vi "trial 1.vi"() -> ()   [LabVIEW 2013]
panel:
  out "number":i32[](array[numeric])
  out "Array 3":i32[][](array[numeric])
  in  "index":i32
  out "Array 2":i32[][](array[numeric])
  in  "Full transition sequence from service to end":string[](array[string])=["-2 0 3 0 -3 0 4 -4 0\r\n", "0 3\r\n", "0 4 -3 0 -4 1 0 4 -3 0\r\n", "0\r\n", "-2 0 3 -3 0 -4 1 -4 0 3 -3 4 -3 0 2 0 3\r\n", "0 3 0 1\r\n", "0 1 0 3\r\n", "0 3 -2 0 4\r\n", "0\r\n", "0 -3 4 0 2 -2 0 -3 0 3 -2 3 -3 4\r\n", "0 -3 4 -3 0\r\n", "-2 0 -2 2 0\r\n", "0 3 -2\r\n", "0 4 -3 0 3 -2 0 -3 4 -3 0 3 -2 2 -2 0 4 0\r\n", "2 0 1 -4 0 3 0 -4 4 0 -4 4 0 2 0 4 0 -3 4 -3 0 -4 0 4\r\n", "0 4\r\n", "-2 0 -2 0 3 0\r\n", "0 3 0 -2 3\r\n", "0 4 0 4 -4 0 2 0 -4 4 -3 0 -2 2 -2 0 4 -3 0 2 0 3 0\r\n", "0 4 -3 0 1 -1 0 3 0 -2 2 -2 0 -3 4 -3 0 4 -4 1 0\r\n", "", "0 -3\r\n", "2 0 3 0 1 0 -2 3\r\n", "0\r\n", "1 -1 0\r\n", "0 -2 3 0\r\n", "0 1 0 4 0 4 -4 4\r\n", "0 1 -1 0 3\r\n", "0 2 -2 3 -3 4\r\n", "-2 2 0 -2 3\r\n", "0 -1\r\n", "0 4 -4 4 0 3 0 -2 0 -4 0 1 -4\r\n", "-2 0 4 0 -3 3 0 -2 2 -2 0 -4 0 4 0\r\n", "0 -1 0 -4 4 -4 1 -4 0\r\n", "1 -4 1 0 2 0 -3 0 2 0 -2 0 1 0 1 -4 4 -4 1 0 3 -2 0 -4 4 -4\r\n", "0 1 -4 4 -4 1\r\n", "0 3 0 -3 3 0 1 0 1 -4 4\r\n", "0 1 -4 0 1 -4\r\n", "0 3 -2 0 1 -4 1 0 2 0 4 0 4 0 -1 2 -1 0\r\n", "1 0 -1 0 2 0 4 -4\r\n", "-4\r\n", "-1 0 4\r\n", "0 1 -1 0 1 -4 0\r\n", "-1 0 1 -4 0 3 0 2 0 4 0 -4 4 -4 0 -1 0 -4 0 -2 0 4\r\n", "0 4 0\r\n", "0 4 -4 0 2 -1 0 2 0 4 -4 1 -4 4 0 3\r\n", "0 4 0 2 0\r\n", "1 0 -1 1 0 -4 1 -4 1 0 -4\r\n", "0 3 -2 0 -4\r\n", "2 -1 0 -4 4 -4 0 2 0 4\r\n", "1 0\r\n", "-1 0 -1 1 0 -4\r\n", "0 3 0\r\n", "0 -4 4 -4 0 -4 0 4 0 2 0 1 -4 4\r\n", "-1 0 1 -4\r\n", "-1 0 2 -1 0 2\r\n", "1 -1 0 4 -4 1\r\n", "-1 0 1 -4 4 -4 0 -4 4\r\n", "0 3 0 3 0 1 -1 0 1\r\n", "-1 0 4 0 4 -4 1 0 -4 0\r\n", "1 0 4\r\n", "0 -1 0 2 -1 0 -2 3 -2 0 -4 4 -4\r\n", "0 3 0\r\n", "2 -1 0 1 -4 4 -4 0 2 0\r\n", "0 4 -4 1 0 1 0 1 -4 0 2 0 4 0 4 -4 1\r\n", "1 -1 0 3 0 3 0 1 0 4\r\n", "0 -4 0 -2 0 -4\r\n", "0 -4 4 -4 0 -2 0 2 0\r\n", "-1 0 4 -4 0\r\n", "1 0 -1 2 0 4\r\n", "0 2 0 -2 0\r\n", "0 1 -4 0 -4 0 3 -2 0 -4 0 -4 4 -4 1\r\n", "0 4 0 4 0 4 0 4 0 -2 3 0 3 0 4 0\r\n", "-4 -1\r\n", "-2 0 1 0 -4 4\r\n", "0 4\r\n", "-2 2 0 -1 -4 1 0 3 0\r\n", "-1 0 -1 2\r\n", "0 -1 1 0 4 0 3 -2 0 -2 3 -2 0 4 0 -2 2\r\n", "2 -1 0 4\r\n", "0 4 0 2 0 -2 0\r\n", "1 -1 0 3 0 -4 4 -4 0\r\n", "2 -1 0 3 -2 0 -3 0 3 0 -3 0\r\n", "0 4 0 4 -4 1 -1 0 -3 0 1 -4 1 0 4 0 -4 0 -4 4 -4 1\r\n", "0 -4 1 0 -4 4\r\n", "0 4 0 -2 2 -2 2 -2 2\r\n", "-2 2 -1 0 4 0 2 0 4 0 2 -2 0 4\r\n", "1 0 -1 0 -1 0 1 -1\r\n", "-2 2 -2 3\r\n", "1 0 -1 0 -1 2 0 2 -2 0 -4 0\r\n", "-2 2 0 3 -2 2\r\n", "0\r\n", "1 -1 0 3\r\n", "0 4 0\r\n", "-2 0 1 -4 0 -3 0\r\n", "1 0 -1 2 -1 1 -4\r\n", "0 4\r\n", "-2 0 -1 1\r\n", "0 3 0 3 0 3 -2\r\n", "-4 0 -4 4\r\n", "0 4 0 -4 0 -4\r\n", "-2 2 0 4 -4 0 2 -2\r\n", "-2 2 -2 0 -1\r\n", "0 4 -3 0\r\n", "0 1 0 -1 1\r\n", "-4 0\r\n", "-2 0 3 0 1 0 3 -2 0 -1 0 4 0 3 0 -3 3 -3\r\n", "0 4 0 -2 0 1 0 -4 4 -3 0 1 0 4 0 -4 1 0 3 -3 0\r\n", "0 -1 2\r\n", "2 0 -3 4 0\r\n", "-4 0 -3 3 -3 0 -3 3 0 -2 3 0\r\n", "0 -1 1 -4 4 -3 0 3 0\r\n", "0 -1 2 0 3 0 1 -4 4 0 2 0\r\n", "2 -2 0 -4 0 -4 4 0 -4\r\n", "1 -1 2 -1\r\n", "2 0 -2 0 4 0 2 0 3 0 -2 0 -4\r\n", "1 -1 0 -1\r\n", "0 1 -4 1\r\n", "0 4 0 -1 1 -1 0\r\n", "0 3\r\n", "-2 0\r\n", "1 -4 0 -2 0 4 0 -4 0 4 -3 0 1 -4 0 1\r\n", "0 -3 3 -2 0 3 0 -2 2\r\n", "1 0\r\n", "2\r\n", "0 -4\r\n", "0 4 0 -4 0 -3 3 -3 0 -2 0 -2 0 4 0 -1 1 0 3 0 -4 1 -4 0 4\r\n", "2 0 -1 1\r\n", "0 2 0 4 0 4 -4 0 -1 2\r\n", "0 3 -2 0 3 -2\r\n", "1 0 -3 3 0 -4\r\n", "0 -3 3 0 -1 0\r\n", "2 -2 0 1\r\n", "-4 1 -4 1 -4 0\r\n", "0 4 0 2 0 -4 1 2 -1 0 4 0 1 0 4 -4 4 0 -4 4 0\r\n", "-2 0 3 0 -2 0\r\n"]
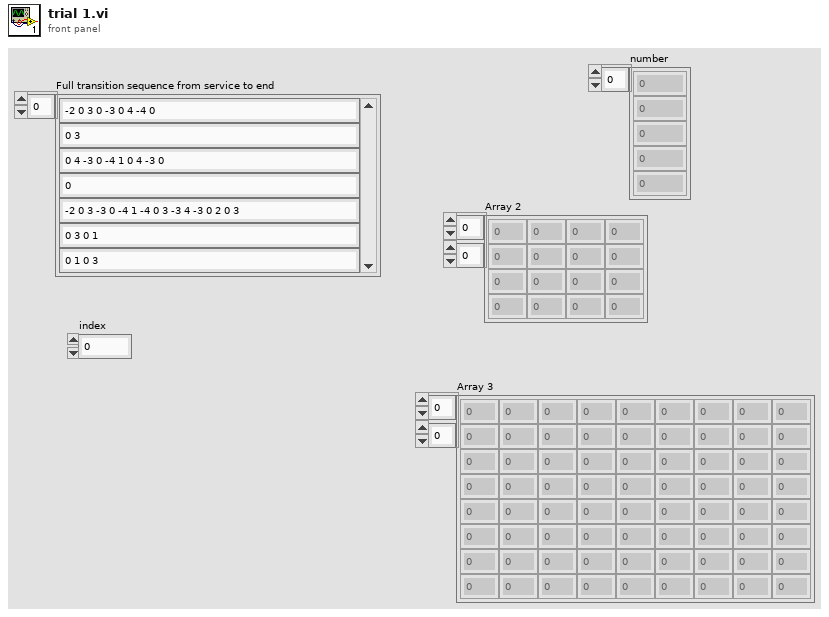
[diagram p1: front panel]
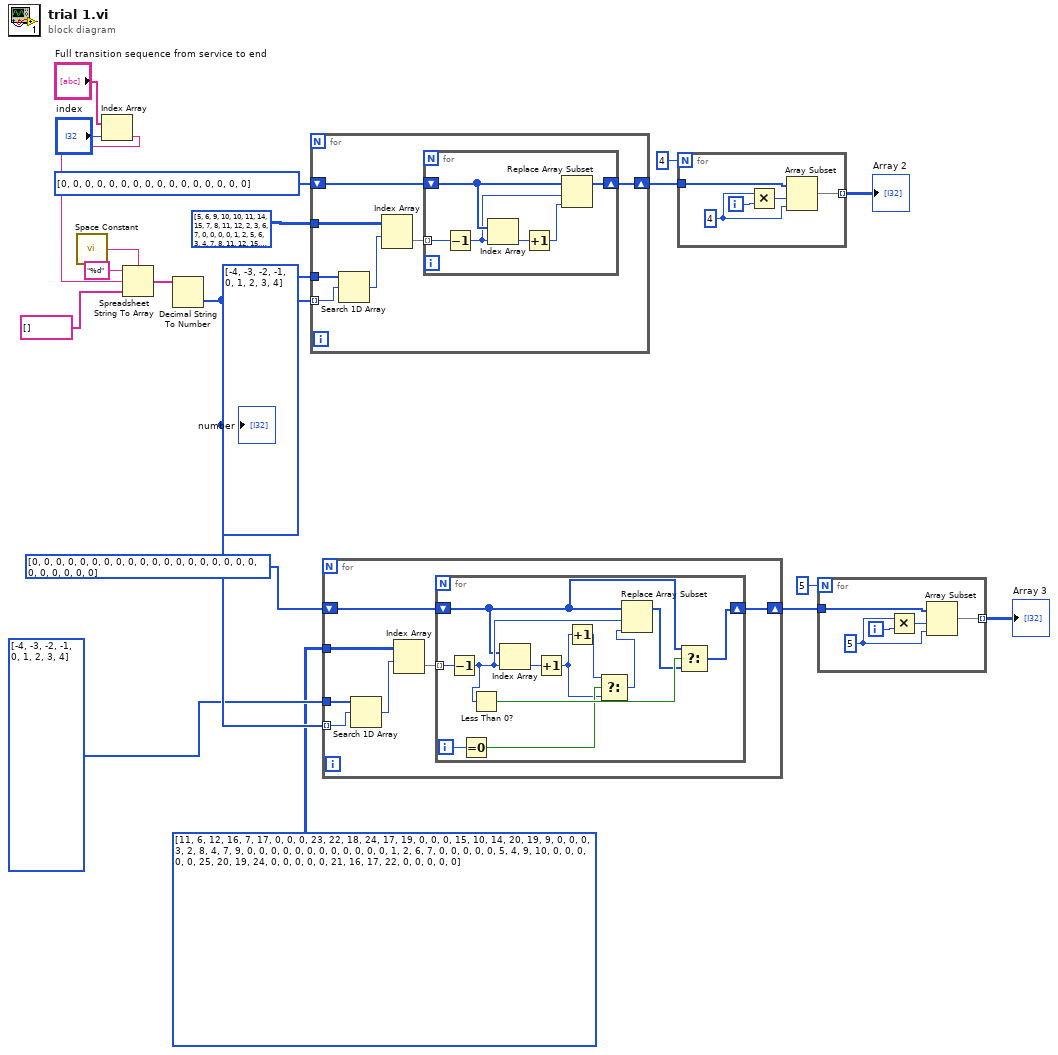
[diagram p0: block diagram]
diagram:
  n1 = call <vilib>:"Space Constant.vi"() -> ("String"=w20:string)
  n2 = Index Array(array="Full transition sequence from service to end", index="index") -> (element=w9:string)
  n3 = Spreadsheet String To Array(delimiter (Tab)=w20, format string="%d", spreadsheet string=w9, array type (2D Dbl)=string[] []) -> (array=w17:string[])
  n4 = Decimal String To Number(string=w17) -> (number=w4:i32[])  [unwired: 2 in, 1 out]
  "number" <- w4
  n5 = for {
    tunnel: w4 -> [w26] mode=indexing
    tunnel: i32[] [-4, -3, -2, -1, 0, 1, 2, 3, 4] ("deleted portion") -> [w27]
    tunnel: i32[][] [[5, 6, 9, 10], [10, 11, 14, 15], [7, 8, 11, 12], [2, 3, 6, 7], [0, 0, 0, 0], [1, 2, 5, 6], [3, 4, 7, 8], [11, 12, 15, 16], [9, 10, 13, 14]] ("array w/ subset deleted") -> [w25]
    shift-right: [w21] -> w13
    shift-left: i32[] [0, 0, 0, 0, 0, 0, 0, 0, 0, 0, 0, 0, 0, 0, 0, 0] -> [w22]
    n6 = Search 1D Array(1D array=w27, element=w26) -> (index of element=w24:i32)  [unwired: 1 in]
    n7 = Index Array(array=w25, index (row)=w24) -> (element=w23:i32[])  [unwired: 1 in]
    n8 = for {
      tunnel: w23 -> [w29] mode=indexing
      shift-right: [w30] -> w21
      shift-left: w22 -> [w32]
      n9 = Decrement(x=w29) -> (x-1=w28:i32)
      n10 = Index Array(array=w32, index=w28) -> (element=w33:i32)
      n11 = Increment(x=w33) -> (x+1=w31:i32)
      n12 = Replace Array Subset(array=w32, new element=w31, index=w28) -> (w30:i32[])
    }
  }
  n13 = for {
    tunnel: w4 -> [w39] mode=indexing
    tunnel: i32[] [-4, -3, -2, -1, 0, 1, 2, 3, 4] ("deleted portion") -> [w40]
    tunnel: i32[][] [[11, 6, 12, 16, 7, 17, 0, 0, 0], [23, 22, 18, 24, 17, 19, 0, 0, 0], [15, 10, 14, 20, 19, 9, 0, 0, 0], [3, 2, 8, 4, 7, 9, 0, 0, 0], [0, 0, 0, 0, 0, 0, 0, 0, 0], [1, 2, 6, 7, 0, 0, 0, 0, 0], [5, 4, 9, 10, 0, 0, 0, 0, 0], [25, 20, 19, 24, 0, 0, 0, 0, 0], [21, 16, 17, 22, 0, 0, 0, 0, 0]] ("array w/ subset deleted") -> [w38]
    shift-right: [w34] -> w5
    shift-left: i32[] [0, 0, 0, 0, 0, 0, 0, 0, 0, 0, 0, 0, 0, 0, 0, 0, 0, 0, 0, 0, 0, 0, 0, 0, 0] -> [w35]
    n14 = Search 1D Array(1D array=w40, element=w39) -> (index of element=w37:i32)  [unwired: 1 in]
    n15 = Index Array(array=w38, index (row)=w37) -> (element=w36:i32[])  [unwired: 1 in]
    n16 = for {
      tunnel: w36 -> [w51] mode=indexing
      shift-right: [w45] -> w34
      shift-left: w35 -> [w47]
      i -> [w50]
      n17 = Decrement(x=w51) -> (x-1=w49:i32)
      n18 = Equal To 0?(x=w50) -> (x = 0?=w44:bool)
      n19 = Less Than 0?(x=w49) -> (x < 0?=w48:bool)
      n20 = Index Array(array=w47, index=w49) -> (element=w52:i32)
      n21 = Increment(x=w52) -> (x+1=w42:i32)
      n22 = Increment(x=w42) -> (x+1=w41:i32)
      n23 = Select(t=w41, s=w44, f=w42) -> (s? t:f=w43:i32)
      n24 = Replace Array Subset(array=w47, new element=w43, index=w49) -> (w46:i32[])
      n25 = Select(t=w47, s=w48, f=w46) -> (s? t:f=w45:i32[])
    }
  }
  n26 = for {
    N: 4 -> [_]
    tunnel: w13 -> [w57]
    tunnel: [w53] -> w11 mode=indexing
    i -> [w56]
    w55 = 4 ("length")
    n27 = Multiply(x=w55, y=w56) -> (x*y=w54:i32)
    n28 = Array Subset(array=w57, index=w54, length=w55) -> (w53:i32[])
  }
  "Array 2" <- w11
  n29 = for {
    N: 5 -> [_]
    tunnel: w5 -> [w62]
    tunnel: [w58] -> w7 mode=indexing
    i -> [w61]
    w60 = 5 ("length")
    n30 = Multiply(x=w60, y=w61) -> (x*y=w59:i32)
    n31 = Array Subset(array=w62, index=w59, length=w60) -> (w58:i32[])
  }
  "Array 3" <- w7
